vi "Radau5_Jacobian Matrix.vi"(0 "Y(k)":dbl[](array[numeric]), 1 "do Jac?":bool, 2 "Step size":dbl, 5 "Y'":dbl[](array[numeric]), 7 "Fout":dbl[](array[numeric]), 9 "Matrix J":T1, 11 "Matrix M":T1, 12 "ErrorTolerance":dbl[](array[numeric])) -> (4 "Ready":bool, 6 "Y(k)":dbl[](array[numeric]), 8 "Y'":dbl[](array[numeric]), 10 "Matrix J":T1, 15 "Matrix M":T1)   [LabVIEW 2020, in "NI_DAE.lvlib"]
uses:
  <vilib>/gmath/NI_DAE.lvlib
  <vilib>/Analysis/Matrix/Datatypes/RealMatrix.ctl
  <vilib>/gmath/dae.llb/Radau5_Jacobian Status.ctl
  <vilib>/gmath/dae.llb/Radau5_Callback Status.ctl
  <vilib>/Analysis/Matrix/NI_Matrix.lvlib
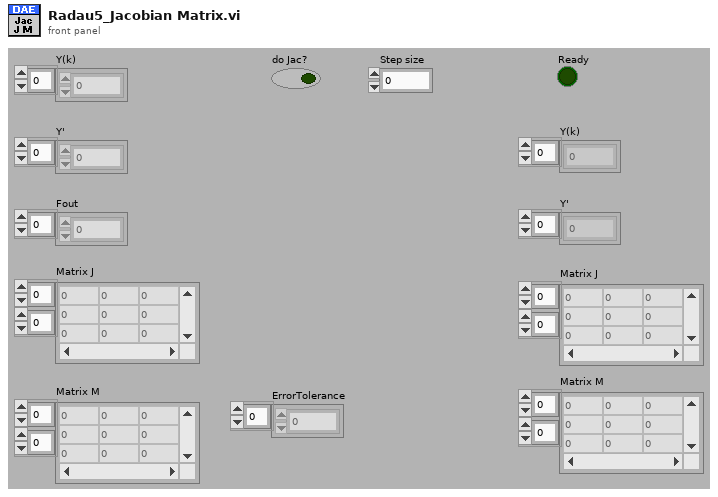
[diagram p1: front panel]
types:
  T1 = typedef "NI_Matrix.lvlib/RealMatrix.ctl" = dbl[][]
  T2 = typedef "NI_DAE.lvlib/Radau5_Jacobian Status.ctl" = enum16{"Calc Matrix J", "Calc Matrix M"}
  T3 = typedef "NI_DAE.lvlib/Radau5_Callback Status.ctl" = enum16{"Before callback", "After callback"}
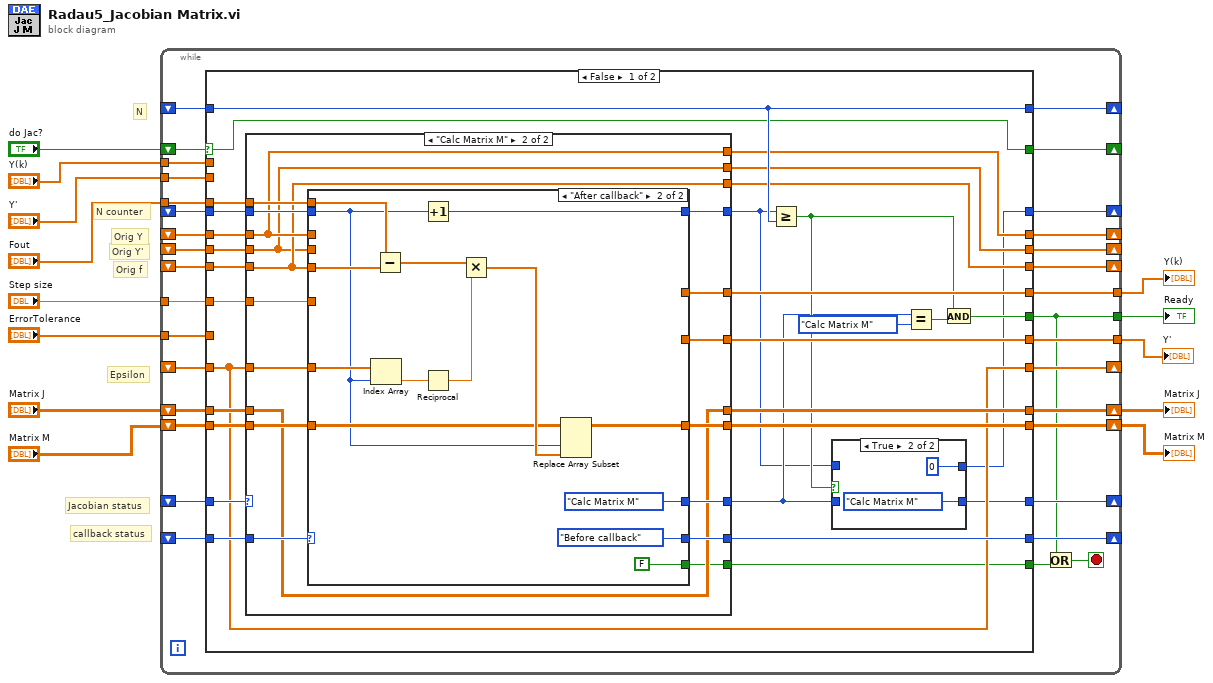
[diagram p0: block diagram]
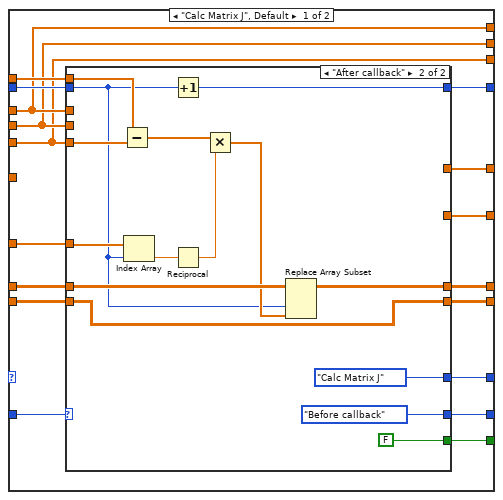
[diagram p3: hidden frame]
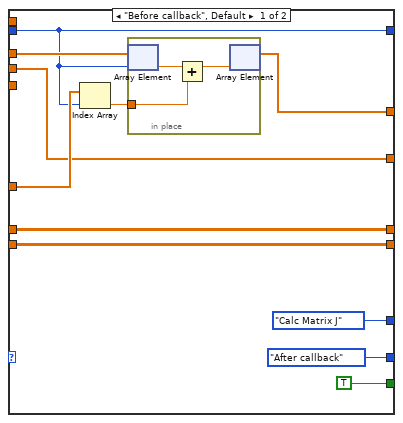
[diagram p4: hidden frame]
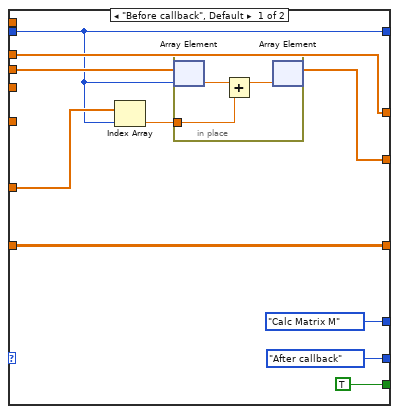
[diagram p5: hidden frame]
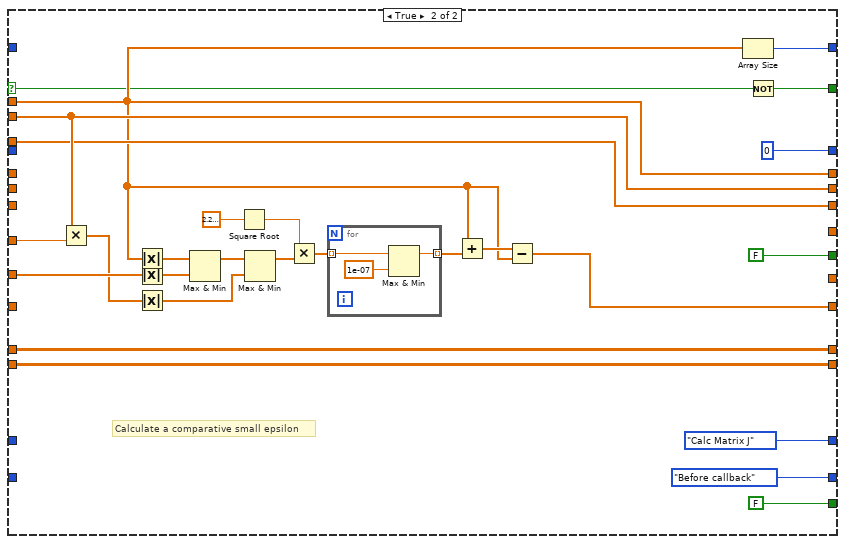
[diagram p6: hidden frame]
diagram:
  # "Orig f"
  # "Jacobian status"
  # "callback status"
  # "N"
  # "N counter"
  # "Orig Y'"
  # "Orig Y"
  # "Epsilon"
  n1 = while {
    shift-right: [w44] -> _
    shift-left: _ -> [w43]
    shift-right: [w42] -> _
    shift-left: _ -> [w41]
    shift-right: [w40] -> _
    shift-left: _ -> [w39]
    tunnel: "Y(k)" -> [w38]
    tunnel: "Y'" -> [w37]
    shift-right: [w35] -> _
    shift-left: _ -> [w34]
    shift-right: [w36] -> _
    shift-left: _ -> [w33]
    tunnel: "Fout" -> [w32]
    tunnel: "ErrorTolerance" -> [w31]
    tunnel: "Step size" -> [w30]
    shift-right: [w29] -> _
    shift-left: _ -> [w28]
    shift-right: [w27] -> _
    shift-left: _ -> [w26]
    shift-right: [w21] -> _
    shift-left: _ -> [w20]
    tunnel: [w19] -> w13
    tunnel: [w18] -> w12
    tunnel: [w17] -> w9
    shift-right: [w14] -> _
    shift-left: "do Jac?" -> [w45]
    shift-right: [w22] -> w10
    shift-left: "Matrix M" -> [w23]
    shift-right: [w24] -> w11
    shift-left: "Matrix J" -> [w25]
    stop <- w16 stop-if-true
    n2 = case shown="False" w45 {
      selector: w45 -> [w49 w173]
      tunnel: [w62 Radau5_Callback_Status."Before callback" ("Callback status")] -> w44
      tunnel: w43 -> [w74 _]
      tunnel: [w54 Radau5_Jacobian_Status."Calc Matrix J" ("Jacobian status")] -> w42
      tunnel: w41 -> [w75 _]
      tunnel: [w47 0] -> w40
      tunnel: w39 -> [w72 _]
      tunnel: w38 -> [_ w174]
      tunnel: w37 -> [_ w184]
      tunnel: [w52 w184] -> w36
      tunnel: [w53 w174] -> w35
      tunnel: w34 -> [w73 _]
      tunnel: w33 -> [w70 _]
      tunnel: w32 -> [w64 w178]
      tunnel: w31 -> [_ w185]
      tunnel: w30 -> [w46 w183]
      tunnel: [w61 w182] -> w29
      tunnel: w28 -> [w61 _]
      tunnel: [w60 w181] -> w27
      tunnel: w26 -> [w60 _]
      tunnel: w25 -> [w68 w180]
      tunnel: [w66 w180] -> w24
      tunnel: w23 -> [w67 w179]
      tunnel: [w65 w179] -> w22
      tunnel: [w51 w178] -> w21
      tunnel: w20 -> [w63 _]
      tunnel: [w71 _] -> w19
      tunnel: [w69 _] -> w18
      tunnel: [w58 FALSE] -> w17
      tunnel: [w50 FALSE] -> w15
      tunnel: [w49 w172] -> w14
      frame False {
        n3 = case shown="\"Calc Matrix M\"" w75 {
          tunnel: w74 -> [w96 w140]
          tunnel: w73 -> [w83 w130]
          tunnel: w72 -> [w95 w138]
          tunnel: [w94 w134] -> w48
          tunnel: w61 -> [w93 w139]
          tunnel: [w92 w136] -> w71
          tunnel: w70 -> [w82 w127]
          tunnel: [w91 w137] -> w69
          tunnel: w68 -> [w90 w131]
          tunnel: w67 -> [w89 w133]
          tunnel: [w88 w131] -> w66
          tunnel: [w87 w132] -> w65
          tunnel: w64 -> [w86 w135]
          tunnel: w63 -> [w81 w129]
          tunnel: [w85 w142] -> w55
          tunnel: [w84 w141] -> w62
          tunnel: [w83 w130] -> w53
          tunnel: [w82 w127] -> w52
          tunnel: [w81 w129] -> w51
          tunnel: [w80 w128] -> w50
          tunnel: w46 -> [_ w126]
          frame "Calc Matrix J", Default {
            n4 = case shown="\"After callback\"" w96 {
              tunnel: w83 -> [w107 _]
              tunnel: [w105 w125] -> w94
              tunnel: w95 -> [w105 w116]
              tunnel: w93 -> [w106 w122]
              tunnel: [w104 _] -> w92
              tunnel: w82 -> [w98 _]
              tunnel: [w98 _] -> w91
              tunnel: w90 -> [w103 w118]
              tunnel: w89 -> [w102 w114]
              tunnel: [w103 w115] -> w88
              tunnel: [w102 w114] -> w87
              tunnel: w86 -> [_ w124]
              tunnel: w81 -> [_ w123]
              tunnel: [Radau5_Jacobian_Status."Calc Matrix J" ("Jacobian status") Radau5_Jacobian_Status."Calc Matrix J" ("Jacobian status")] -> w85
              tunnel: [Radau5_Callback_Status."After callback" ("Callback status") Radau5_Callback_Status."Before callback" ("Callback status")] -> w84
              tunnel: [TRUE FALSE] -> w80
              frame "Before callback", Default {
                n5 = Index Array(array=w106, index=w105) -> (element=w97:dbl)
                n6 = in-place {
                  in-place-border: w97 -> [w109]
                  n7 = in-place-array #1(w107, w105) -> (w110:dbl)
                  n8 = Add(x=w110, y=w109) -> (x+y=w108:dbl)
                  n9 = in-place-array #1(w108) -> (w104:dbl[])  [unwired: 1 out]
                }
              }
              frame "After callback" {
                n10 = Subtract(x=w124, y=w123) -> (x-y=w120:dbl[])
                n11 = Index Array(array=w122, index=w116) -> (element=w121:dbl)
                n12 = Increment(x=w116) -> (x+1=w125:i32)
                n13 = Reciprocal(x=w121) -> (1/x=w119:dbl)
                n14 = Multiply(x=w120, y=w119) -> (x*y=w117:dbl[])
                n15 = Replace Array Subset(array=w118, new element=w117, index (col)=w116) -> (w115:T1)  [unwired: 1 in]
              }
            }
          }
          frame "Calc Matrix M" {
            n16 = case shown="\"After callback\"" w140 {
              tunnel: [Radau5_Jacobian_Status."Calc Matrix M" ("Jacobian status") Radau5_Jacobian_Status."Calc Matrix M" ("Jacobian status")] -> w142
              tunnel: [Radau5_Callback_Status."After callback" ("Callback status") Radau5_Callback_Status."Before callback" ("Callback status")] -> w141
              tunnel: w139 -> [w150 w163]
              tunnel: w138 -> [w145 w158]
              tunnel: w127 -> [w149 _]
              tunnel: [w148 _] -> w137
              tunnel: w130 -> [w147 _]
              tunnel: [w147 _] -> w136
              tunnel: w135 -> [_ w165]
              tunnel: w129 -> [_ w164]
              tunnel: [w145 w162] -> w134
              tunnel: w133 -> [w146 w159]
              tunnel: [w146 w157] -> w132
              tunnel: [TRUE FALSE] -> w128
              tunnel: w126 -> [_ _]
              frame "Before callback", Default {
                n17 = Index Array(array=w150, index=w145) -> (element=w143:dbl)
                n18 = in-place {
                  in-place-border: w143 -> [w153]
                  n19 = in-place-array #2(w149, w145) -> (w155:dbl)
                  n20 = Add(x=w155, y=w153) -> (x+y=w154:dbl)
                  n21 = in-place-array #2(w154) -> (w148:dbl[])  [unwired: 1 out]
                }
              }
              frame "After callback" {
                n22 = Index Array(array=w163, index=w158) -> (element=w161:dbl)
                n23 = Subtract(x=w165, y=w164) -> (x-y=w169:dbl[])
                n24 = Increment(x=w158) -> (x+1=w162:i32)
                n25 = Reciprocal(x=w161) -> (1/x=w168:dbl)
                n26 = Multiply(x=w169, y=w168) -> (x*y=w160:dbl[])
                n27 = Replace Array Subset(array=w159, new element=w160, index (col)=w158) -> (w157:T1)  [unwired: 1 in]
              }
            }
          }
        }
        n28 = Greater Or Equal?(x=w48, y=w60) -> (x >= y?=w57:bool)
        n29 = case shown="True" w57 {
          tunnel: w55 -> [w77 _]
          tunnel: [w77 Radau5_Jacobian_Status."Calc Matrix M" ("Jacobian status")] -> w54
          tunnel: w48 -> [w76 _]
          tunnel: [w76 0] -> w47
          frame False {
          }
          frame True {
          }
        }
        n30 = Equal?(x=w55, y=Radau5_Jacobian_Status."Calc Matrix M" ("Jacobian status")) -> (x = y?=w59:bool)
        n31 = And(x=w57, y=w59) -> (x .and. y?=w58:bool)
      }
      frame True {
        # "Calculate a comparative small epsilon"
        n32 = Multiply(x=w184, y=w183) -> (x*y=w175:dbl[])
        n33 = Absolute Value(x=w174) -> (abs(x)=w191:dbl[])
        n34 = Absolute Value(x=w185) -> (abs(x)=w190:dbl[])
        n35 = Absolute Value(x=w175) -> (abs(x)=w187:dbl[])
        n36 = Max & Min(x=w191, y=w190) -> (max(x,y)=w192:dbl[])  [unwired: 1 out]
        n37 = Square Root(x=2.220446049250313e-16) -> (sqrt(x)=w189:dbl)
        n38 = Max & Min(x=w192, y=w187) -> (max(x,y)=w188:dbl[])  [unwired: 1 out]
        n39 = Multiply(x=w189, y=w188) -> (x*y=w171:dbl[])
        n40 = for {
          tunnel: w171 -> [w199] mode=indexing
          tunnel: [w198] -> w170 mode=indexing
          n41 = Max & Min(x=w199, y=1e-07) -> (max(x,y)=w198:dbl)  [unwired: 1 out]
        }
        n42 = Add(x=w174, y=w170) -> (x+y=w186:dbl[])
        n43 = Subtract(x=w186, y=w174) -> (x-y=w182:dbl[])
        n44 = Array Size(array=w174) -> (size(s)=w181:i32)
        n45 = Not(x=w173) -> (.not. x?=w172:bool)
      }
    }
    n46 = Or(x=w17, y=w15) -> (x .or. y?=w16:bool)
  }
  "Y(k)" <- w13
  "Y'" <- w12
  "Matrix J" <- w11
  "Matrix M" <- w10
  "Ready" <- w9
